vi "tester.vi"() -> ()   [LabVIEW 2015]
panel:
  out "Progress":u8(slide) max=4 scale=0.0..5.0
  in  "Multicolumn Listbox":i32(listbox)
  out "Success":bool
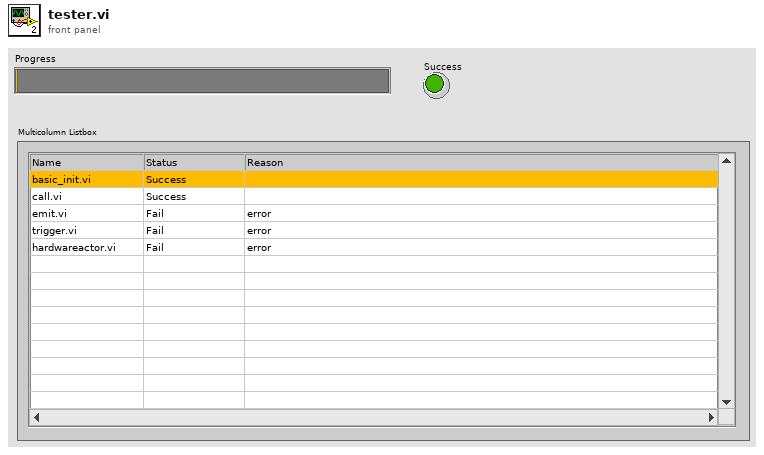
[diagram p1: front panel]
types:
  T1 = typedef "tester_result.ctl" = cluster{"success":bool, "reason":string, "error out":errorcluster}
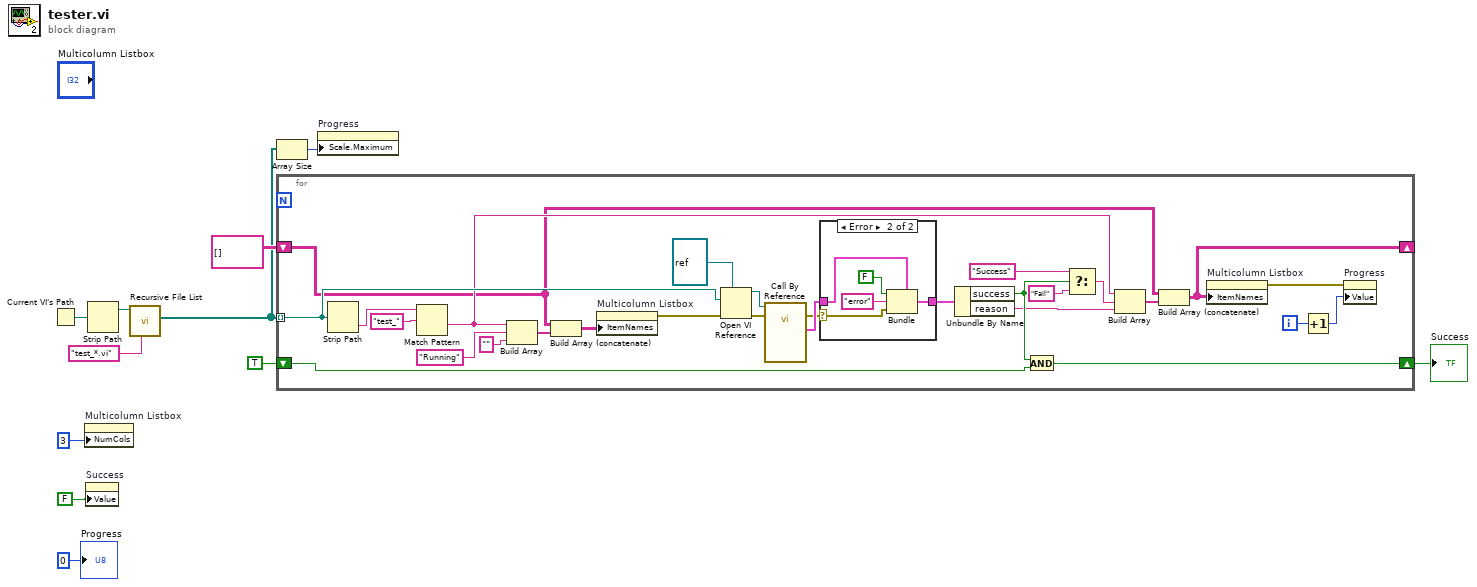
[diagram p0: block diagram]
diagram:
  n1 = Current VI's Path() -> (path=w9:path)
  n2 = property on="Multicolumn Listbox" class="MCListbox (strict)"("NumCols"=u32 3 ("Number of Columns")) -> ()  [unwired: 2 in, 2 out]
  n3 = property on="Success" class="Bool (strict)"("Value"=FALSE ("Success")) -> ()  [unwired: 2 in, 2 out]
  n4 = Strip Path(path=w9) -> (stripped path=w8:path)  [unwired: 1 out]
  n5 = call <vilib>:"Recursive File List.vi"("pattern"="test_*.vi", "Folder Path"=w8) -> ("All Files in Dir"=w2:path[])  [unwired: 5 in, 4 out]
  n6 = Array Size(array=w2) -> (size(s)=w1:i32)
  n7 = for {
    tunnel: w2 -> [w37] mode=indexing
    shift-right: [w34] -> w5
    shift-left: TRUE -> [w33]
    shift-right: [w15] -> _
    shift-left: string[][] [] ("Item Names") -> [w16]
    i -> [w13]
    n8 = Strip Path(path=w37) -> (name=w36:string)  [unwired: 1 out]
    n9 = Match Pattern(string=w36, regular expression="test_") -> (after substring=w23:string)  [unwired: 1 in, 3 out]
    n10 = Build Array(w23, "Running" ("element"), "" ("element")) -> (w25:string[])
    n11 = Build Array (concatenate)(w16, w25) -> (w26:string[][])
    n12 = property on="Multicolumn Listbox" class="MCListbox (strict)"("ItemNames"=w26) -> (error out=w24:errorcluster)  [unwired: 2 in, 1 out]
    n13 = Open VI Reference(type specifier VI Refnum (for type only)=refnum<vi> refnum ("application reference (local)"), vi path=w37, error in (no error)=w24) -> (vi reference=w39:refnum<vi>, error out=w32:errorcluster)  [unwired: 3 in]
    n14 = call-by-ref "?"(reference=w39, error in=w32) -> (error out=w29:errorcluster, "test_result"=w31:T1)  [unwired: 11 in, 1 out]
    n15 = case shown="Error" w29 {
      selector: w29 -> [_ w42]
      tunnel: w31 -> [w40 w45]
      tunnel: [w40 w41] -> w30
      frame No Error {
      }
      frame Error {
        n16 = Bundle(cluster=w45, "success"=FALSE, "reason"="error", "error out"=w42) -> (w41:T1)
      }
    }
    n17 = Unbundle By Name(w30) -> ("success"=w22:bool, "reason"=w18:string)
    n18 = And(x=w22, y=w33) -> (x .and. y?=w34:bool)
    n19 = Select(t="Success" ("element"), s=w22, f="Fail" ("element")) -> (s? t:f=w21:string)
    n20 = Build Array(w23, w21, w18) -> (w17:string[])
    n21 = Build Array (concatenate)(w16, w17) -> (w15:string[][])
    n22 = property on="Multicolumn Listbox" class="MCListbox (strict)"("ItemNames"=w15) -> (error out=w14:errorcluster)  [unwired: 2 in, 1 out]
    n23 = Increment(x=w13) -> (x+1=w12:i32)
    n24 = property on="Progress" class="Slide (strict)"(error in=w14, "Value"=w12) -> ()  [unwired: 1 in, 2 out]
  }
  "Success" <- w5
  n25 = property on="Progress" class="Slide (strict)"("Scale.Maximum"=w1) -> ()  [unwired: 2 in, 2 out]
  "Progress" <- u8 0 ("Progress")
